vi "Making by Hot.vi"(0 "configuration file path":path caption="配置文件的路径", 1 "making by hot msic inf":T1) -> ()   [LabVIEW 2014]
uses:
  Ctl.xio/Making by Hot msic ctl.ctl
  SubVIS.xio/DataSocket/DataSocket_Tags.ctl
  Ctl.xio/part type.ctl
  <vilib>/Utility/file.llb/Read From Spreadsheet File (string).vi
panel:
  in  "SQL information":string
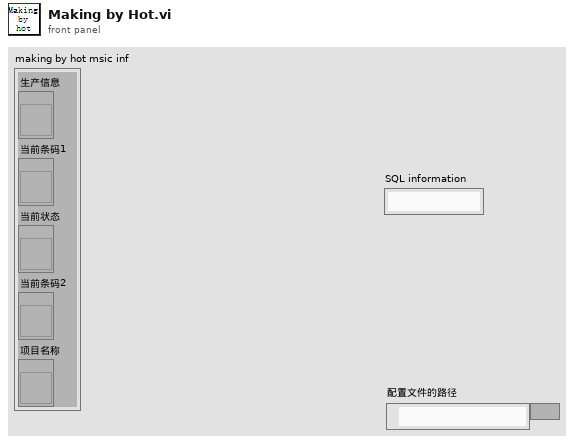
[diagram p1: front panel]
types:
  T1 = cluster{"生产信息":refnum<vi>, "当前条码1":refnum<vi>, "当前状态":refnum<vi>, "当前条码2":refnum<vi>, "项目名称":refnum<vi>}
  T2 = typedef "Making by Hot msic ctl.ctl" = cluster{"configuration file path":path, "DsOut":T3[], "BarCode1":string, "Hopper car information":cluster{"Hopper car code":string, "Hopper car No":string, "plate No":string}, "pallet.produced number":i32, "SQL information":string, "Database":string[], "Serial number":i32, "database path":path, "making by hot msic inf":cluster{"生产信息":refnum<vi>, "当前条码1":refnum<vi>, "当前状态":refnum<vi>, "当前条码2":refnum<vi>, "项目名称":refnum<vi>}, "scnner1 connect id":refnum<k5>, "scnner2 connect id":refnum<k5>, "scanner1 IP":string, "scanner2 IP":string, "BarCode2":string, "Heating process parameters":cluster{"heating start":string, "heating finish":string, "Heating time use":u32}, "part type":T4}
  T3 = typedef "DataSocket_Tags.ctl" = cluster{"Ds ID":refnum<k13>, "Tag":string}
  T4 = typedef "part type.ctl" = cluster{"项目号":string, "物料代码":string, "零件号":string, "供应商编码":string, "产线编码":string, "客户代码":string, "颜色代码":string, "托盘上限":i32, "加热温度":string, "加热时长":string, "EOL Stations":string}
  T5 = cluster{"Hopper car code":string, "Hopper car No":string, "plate No":string}
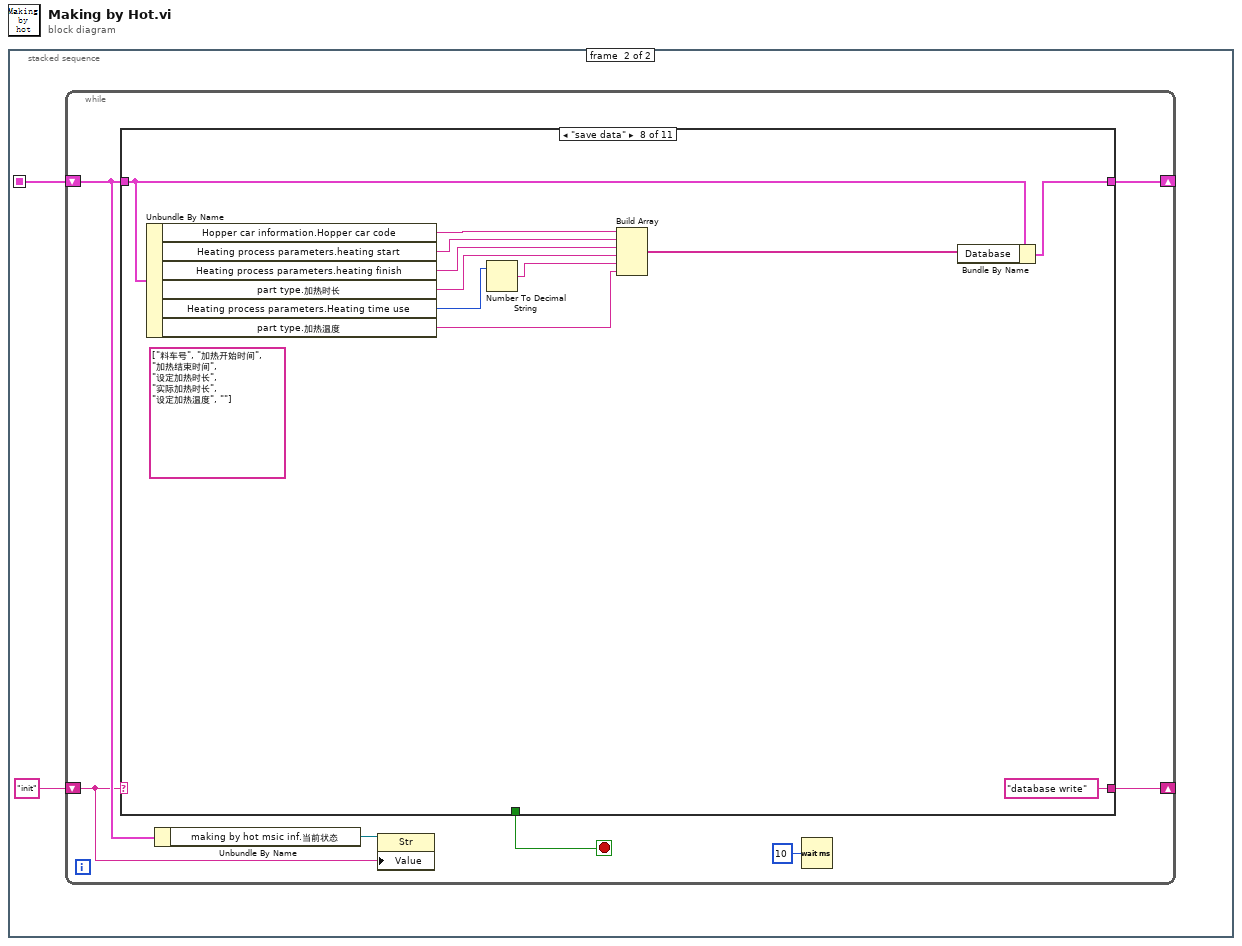
[diagram p0: block diagram]
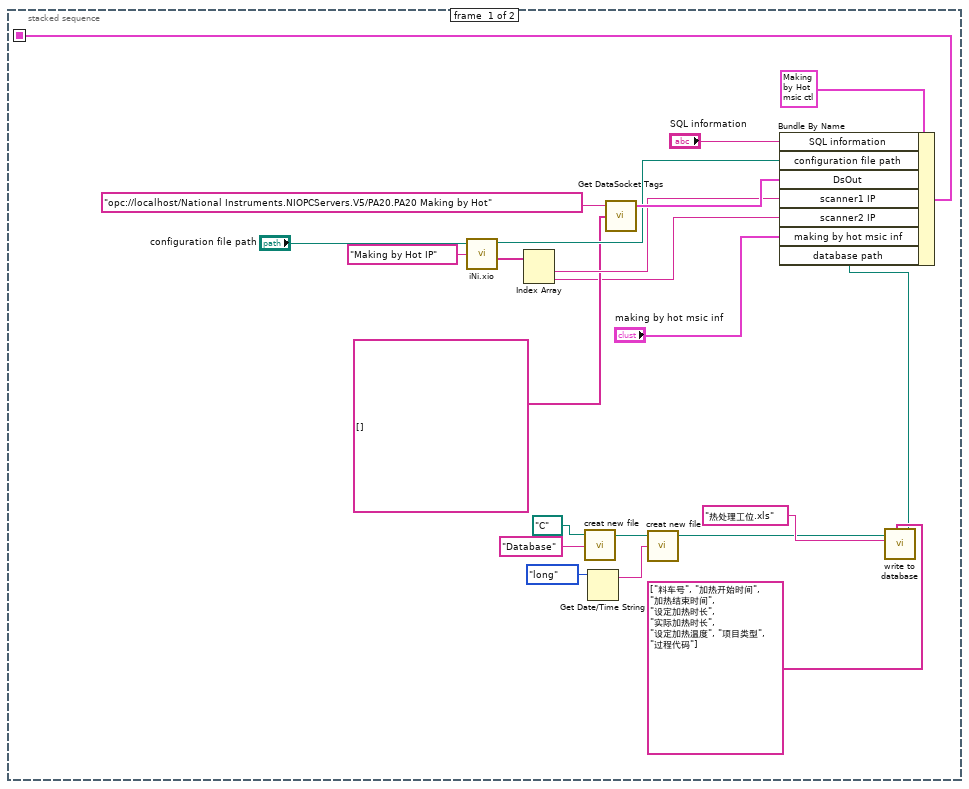
[diagram p2: hidden frame]
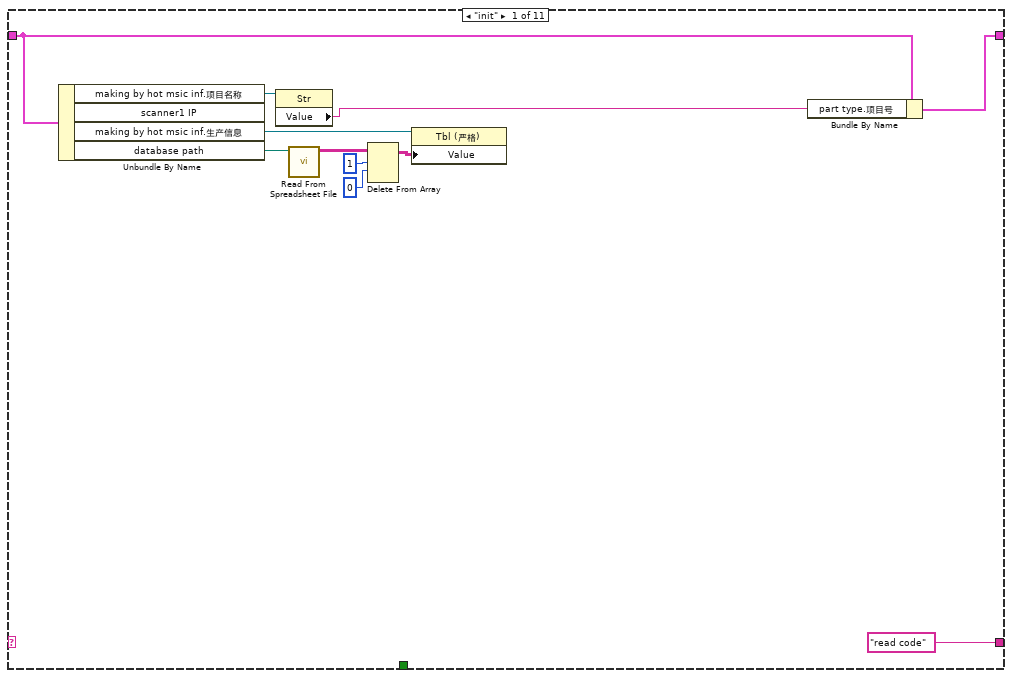
[diagram p3: hidden frame]
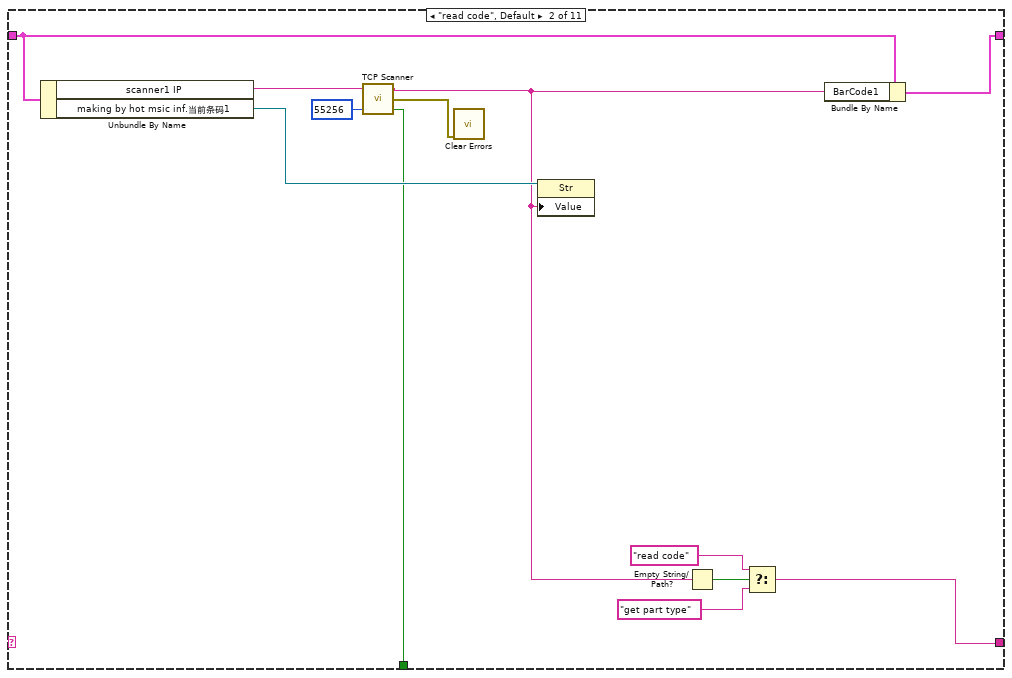
[diagram p4: hidden frame]
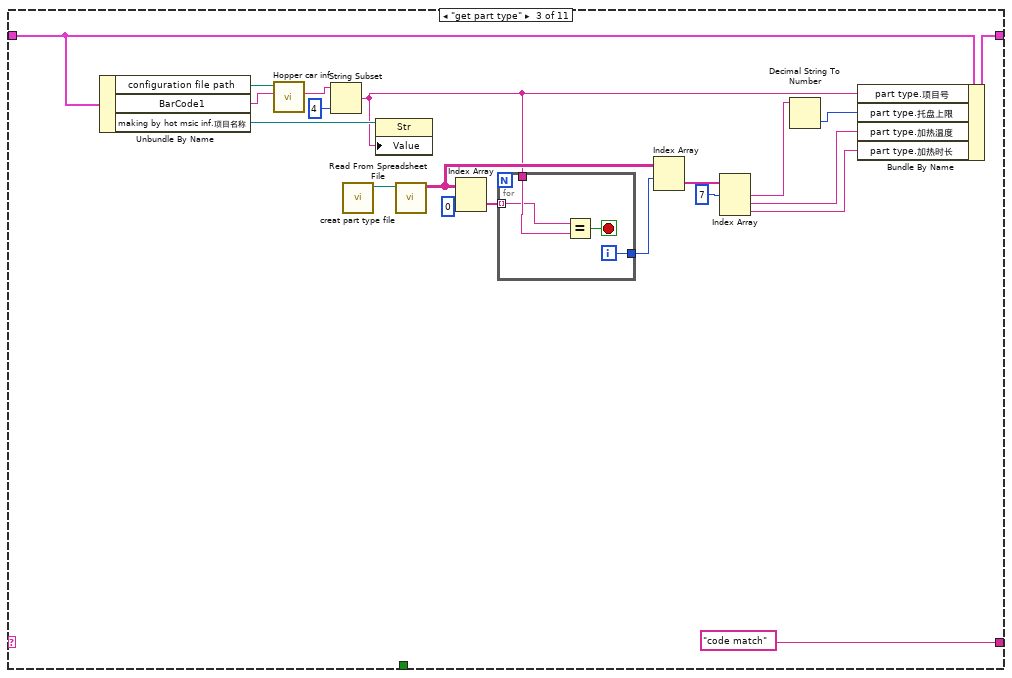
[diagram p5: hidden frame]
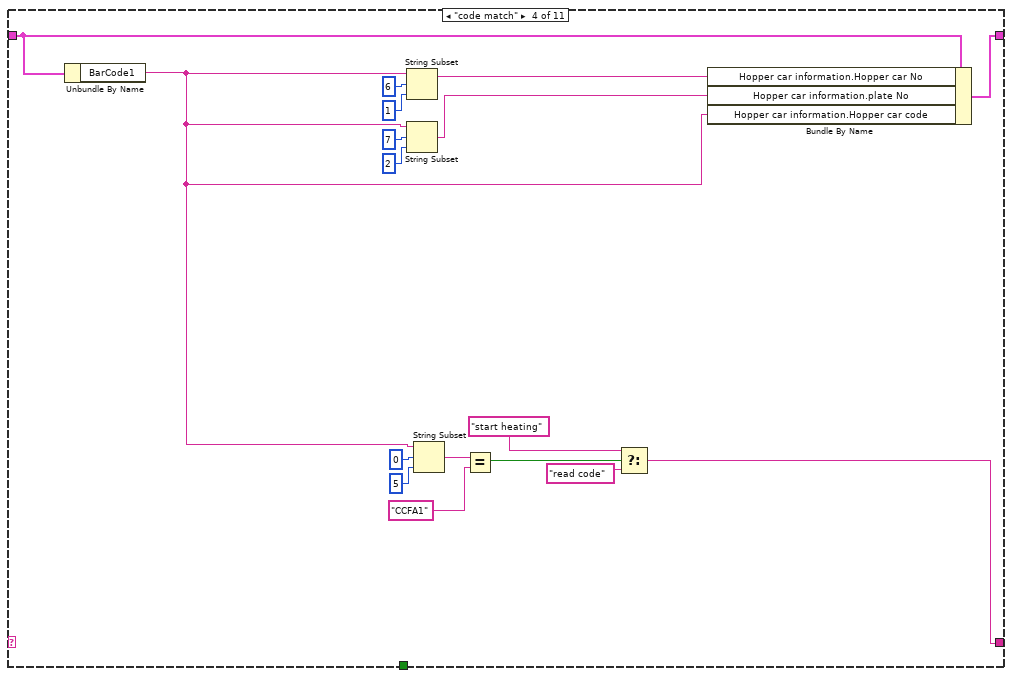
[diagram p6: hidden frame]
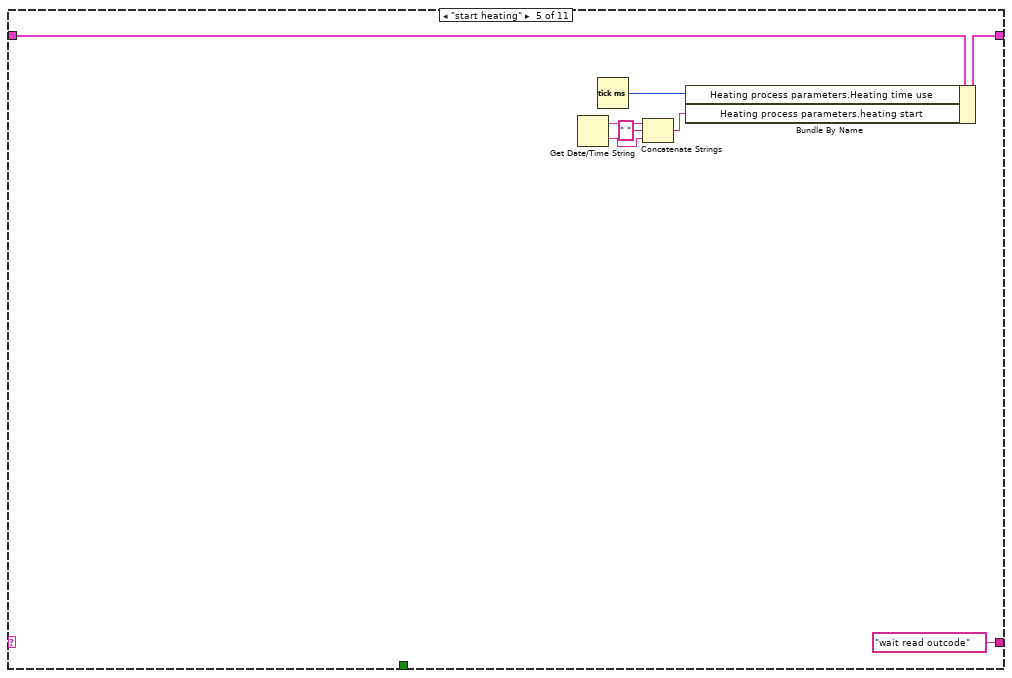
[diagram p7: hidden frame]
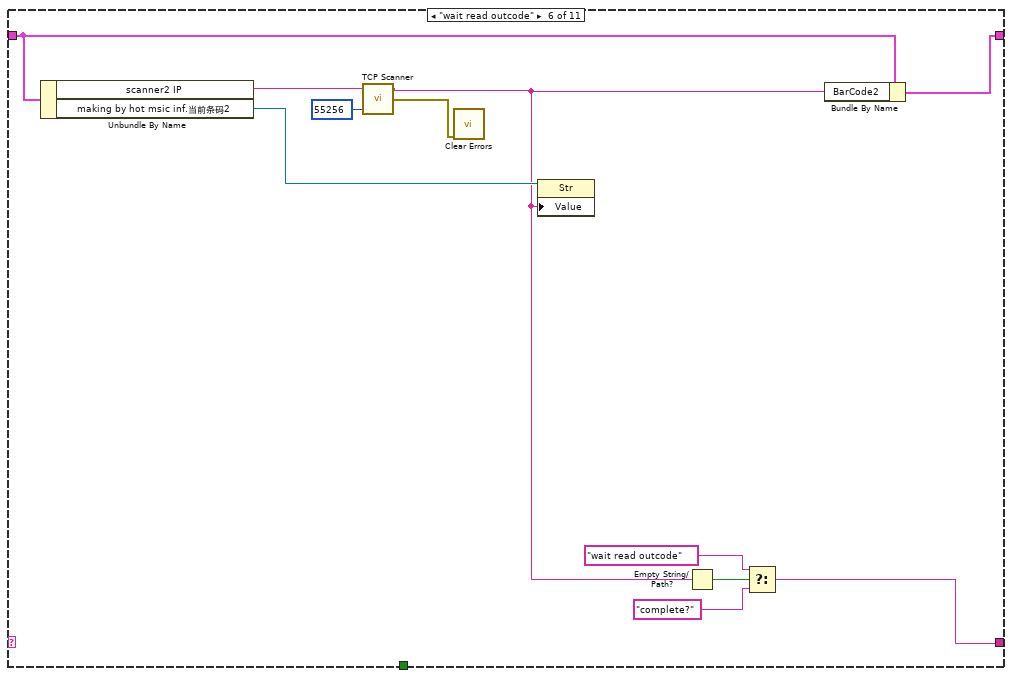
[diagram p8: hidden frame]
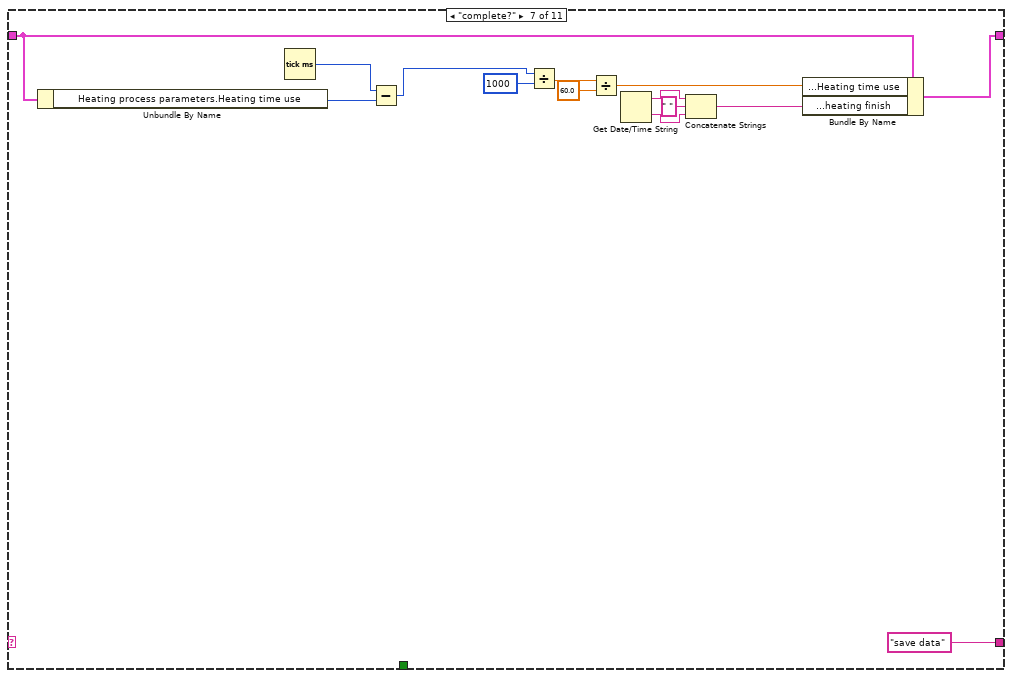
[diagram p9: hidden frame]
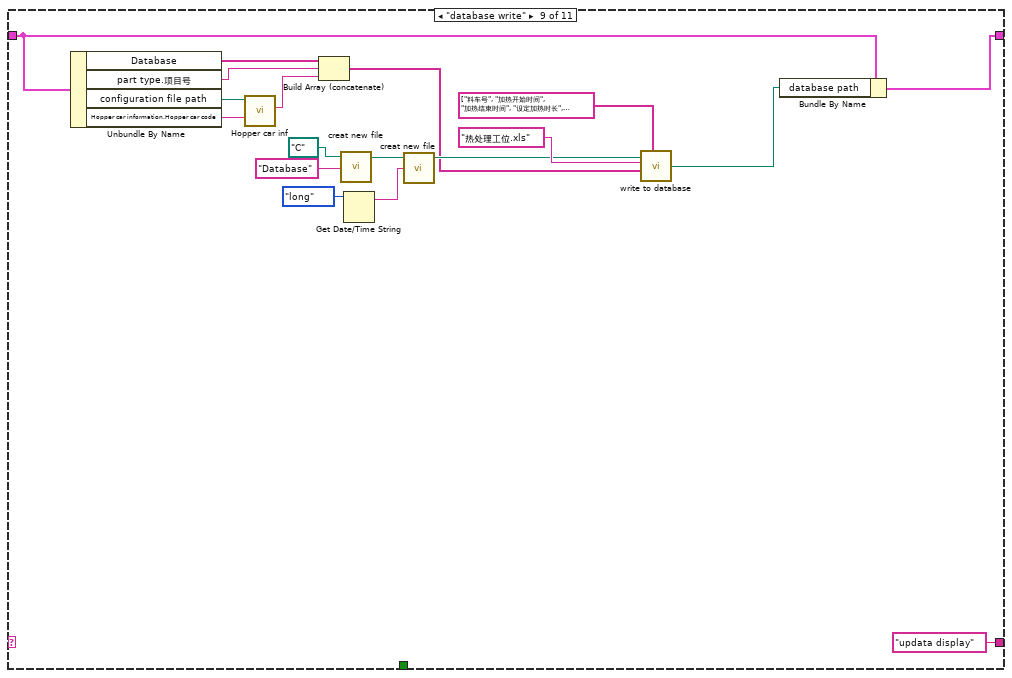
[diagram p10: hidden frame]
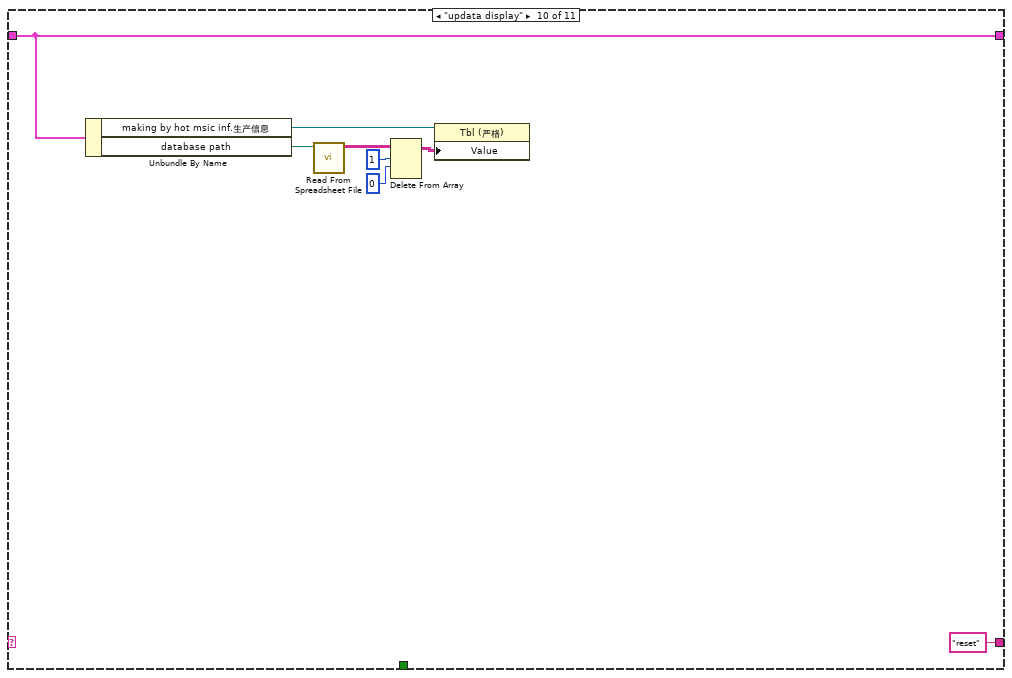
[diagram p11: hidden frame]
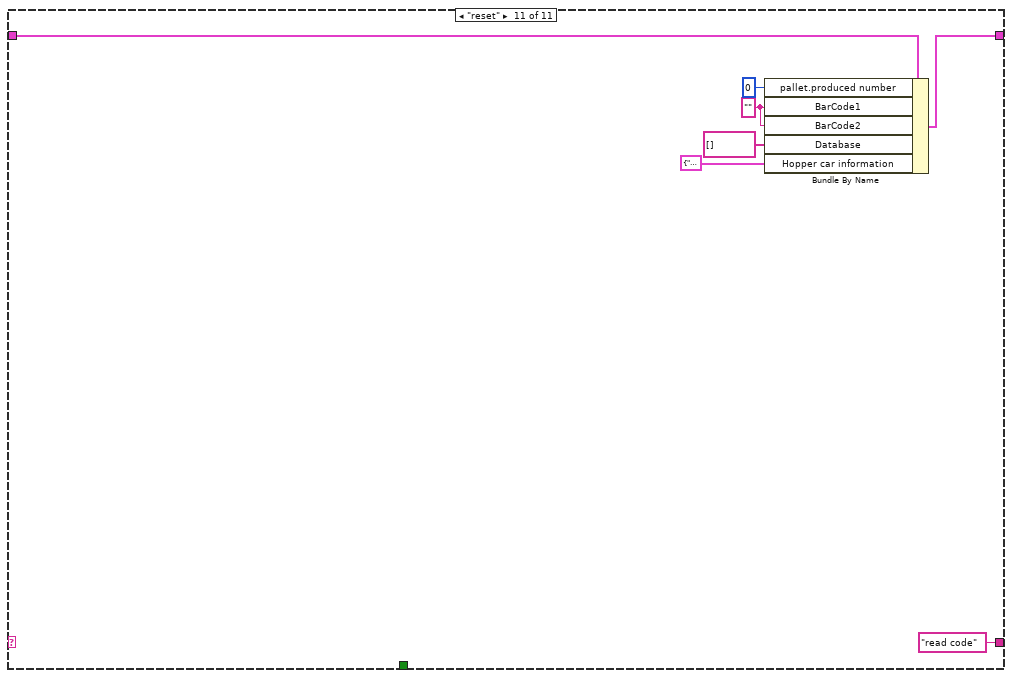
[diagram p12: hidden frame]
diagram:
  n1 = stacked-sequence {
    seq-local: [w10 _] -> [_ w23]
    frame #0 {
      n2 = call "iNi.xio.vi"("configuration file path"="configuration file path", "Sections"="Making by Hot IP") -> ("configuration file path"=w21:path, "Values"=w19:string[])  [unwired: 1 in, 3 out]
      n3 = Index Array(array=w19) -> (element #1=w18:string, element #2=w12:string)  [unwired: 2 in]
      n4 = call "creat new file.vi"("file name"="Database", "path"=path "C:/") -> ("created path"=w5:path)  [unwired: 1 in, 2 out]
      n5 = Get Date/Time String(date format (0)=enum16{"short", "long", "abbreviated"}."long" ("日期格式(0)")) -> (date string=w3:string)  [unwired: 2 in, 1 out]
      n6 = call "Get DataSocket Tags.vi"("All Tags"=string[] [], "URL"="opc://localhost/National Instruments.NIOPCServers.V5/PA20.PA20 Making by Hot") -> ("DsOut"=w22:T3[])  [unwired: 3 in]
      n7 = call "creat new file.vi"("file name"=w3, "path"=w5) -> ("created path"=w4:path)  [unwired: 1 in, 2 out]
      n8 = call "write to database.vi"("Header"=string[] ["料车号", "加热开始时间", "加热结束时间", "设定加热时长", "实际加热时长", "设定加热温度", "项目类型", "过程代码"], "file name"="热处理工位.xls", "path"=w4) -> ("new file path (Not A Path if cancelled)"=w2:path)  [unwired: 3 in]
      n9 = Bundle By Name(cluster=T2 {"configuration file path"=path "", "DsOut"=[], "BarCode1"="", "Hopper car information"={"Hopper car code"="", "Hopper car No"="", "plate No"=""}, "pallet.produced number"=0, "SQL information"="", "Database"=[], "Serial number"=0, "database path"=path "", "making by hot msic inf"={"生产信息"=refnum, "当前条码1"=refnum, "当前状态"=refnum, "当前条码2"=refnum, "项目名称"=refnum}, "scnner1 connect id"=refnum, "scnner2 connect id"=refnum, "scanner1 IP"="", "scanner2 IP"="", "BarCode2"="", "Heating process parameters"={"heating start"="", "heating finish"="", "Heating time use"=0}, "part type"={"项目号"="", "物料代码"="", "零件号"="", "供应商编码"="", "产线编码"="", "客户代码"="", "颜色代码"="", "托盘上限"=0, "加热温度"="", "加热时长"="", "EOL Stations"=""}} ("Making by Hot msic ctl"), "SQL information"="SQL information", "configuration file path"=w21, "DsOut"=w22, "scanner1 IP"=w18, "scanner2 IP"=w12, "making by hot msic inf"="making by hot msic inf", "database path"=w2) -> (w10:T2)
    }
    frame #1 {
      n10 = while {
        shift-right: [w31] -> _
        shift-left: w23 -> [w27]
        shift-right: [w30] -> _
        shift-left: "init" ("event") -> [w26]
        stop <- w25 stop-if-true
        n11 = case shown="\"save data\"" w26 {
          tunnel: w27 -> [w40 w52 w59 w80 w101 w112 w126 w138 w150 w162 w169]
          tunnel: [w42 w54 w74 w89 w103 w114 w121 w129 w151 w162 w171] -> w31
          tunnel: ["read code" w48 "code match" w87 "wait read outcode" ("event") w108 "save data" ("event") "database write" ("f") "updata display" ("f") "reset" ("f") "read code" ("f")] -> w30
          tunnel: [_ w43 _ _ _ _ _ _ _ _ _] -> w25
          frame "init" {
            n12 = Unbundle By Name(w40) -> ("making by hot msic inf.项目名称"=w39:refnum<vi>, "making by hot msic inf.生产信息"=w41:refnum<vi>, "database path"=w36:path)  [unwired: 1 out]
            n13 = property class="Str"(reference=w39) -> ("Value"=w38:string)  [unwired: 1 in, 2 out]
            n14 = call-poly <vilib>:"Read From Spreadsheet File.vi"("file path (dialog if empty)"=w36) -> ("all rows"=w33:string[][])  [unwired: 6 in, 4 out]
            n15 = Delete From Array(array=w33, length=1 ("长度"), index (row)=0 ("索引 (行)")) -> (array with subset deleted=w32:string[][])  [unwired: 1 in, 1 out]
            n16 = property class="Tbl (严格)"(reference=w41, "Value"=w32) -> ()  [unwired: 1 in, 2 out]
            n17 = Bundle By Name(cluster=w40, "part type.项目号"=w38) -> (w42:T2)
          }
          frame "read code", Default {
            n18 = Unbundle By Name(w52) -> ("scanner1 IP"=w46:string, "making by hot msic inf.当前条码1"=w53:refnum<vi>)
            n19 = call "TCP Scanner.vi"("Port（4001）"=u16 55256 ("远程端口或服务名称"), "ip"=w46) -> ("status"=w43:bool, "错误输出"=w44:errorcluster, "Barcode"=w45:string)  [unwired: 1 in]
            n20 = call <vilib>:"Clear Errors.vi"("error in (no error)"=w44) -> ()  [unwired: 5 in, 2 out]
            n21 = property class="Str"(reference=w53, "Value"=w45) -> ()  [unwired: 1 in, 2 out]
            n22 = Empty String/Path?(string/path=w45) -> (empty?=w51:bool)
            n23 = Select(t="read code" ("f"), s=w51, f="get part type") -> (s? t:f=w48:string)
            n24 = Bundle By Name(cluster=w52, "BarCode1"=w45) -> (w54:T2)
          }
          frame "get part type" {
            n25 = Unbundle By Name(w59) -> ("configuration file path"=w61:path, "BarCode1"=w60:string, "making by hot msic inf.项目名称"=w58:refnum<vi>)
            n26 = call "Hopper car inf.vi"("key"=w60, "path in"=w61) -> ("value out"=w57:string)  [unwired: 8 in, 1 out]
            n27 = String Subset(string=w57, length (rest)=4 ("长度（剩余）")) -> (substring=w55:string)  [unwired: 1 in]
            n28 = call "creat part type file.vi"() -> ("new file path (Not A Path if cancelled)"=w63:path)  [unwired: 11 in]
            n29 = property class="Str"(reference=w58, "Value"=w55) -> ()  [unwired: 1 in, 2 out]
            n30 = call-poly <vilib>:"Read From Spreadsheet File.vi"("file path (dialog if empty)"=w63) -> ("all rows"=w70:string[][])  [unwired: 6 in, 4 out]
            n31 = Index Array(array=w70, index (col)=0 ("禁用的索引 (列)")) -> (element=w72:string[])  [unwired: 1 in]
            n32 = for {
              tunnel: w72 -> [w75] mode=indexing
              tunnel: [w77] -> w69
              tunnel: w55 -> [w76]
              i -> [w77]
              stop <- w78 stop-if-true
              n33 = Equal?(x=w75, y=w76) -> (x = y?=w78:bool)
            }
            n34 = Index Array(array=w70, index (row)=w69) -> (element=w68:string[])  [unwired: 1 in]
            n35 = Index Array(array=w68, index #1=7 ("索引")) -> (element #1=w67:string, element #2=w65:string, element #3=w64:string)  [unwired: 2 in]
            n36 = Decimal String To Number(string=w67) -> (number=w66:i32)  [unwired: 2 in, 1 out]
            n37 = Bundle By Name(cluster=w59, "part type.项目号"=w55, "part type.托盘上限"=w66, "part type.加热温度"=w65, "part type.加热时长"=w64) -> (w74:T2)
          }
          frame "code match" {
            n38 = Unbundle By Name(w80) -> ("BarCode1"=w79:string)
            n39 = String Subset(string=w79, offset (0)=6 ("偏移量(0)"), length (rest)=1 ("长度（剩余）")) -> (substring=w82:string)
            n40 = String Subset(string=w79, offset (0)=7 ("偏移量(0)"), length (rest)=2 ("长度（剩余）")) -> (substring=w83:string)
            n41 = String Subset(string=w79, offset (0)=0 ("偏移量(0)"), length (rest)=5 ("长度（剩余）")) -> (substring=w84:string)
            n42 = Equal?(x=w84, y="CCFA1") -> (x = y?=w88:bool)
            n43 = Select(t="start heating" ("event"), s=w88, f="read code" ("event")) -> (s? t:f=w87:string)
            n44 = Bundle By Name(cluster=w80, "Hopper car information.Hopper car No"=w82, "Hopper car information.plate No"=w83, "Hopper car information.Hopper car code"=w79) -> (w89:T2)
          }
          frame "start heating" {
            n45 = Get Date/Time String() -> (date string=w99:string, time string=w97:string)  [unwired: 3 in]
            n46 = Tick Count (ms)() -> (millisecond timer value=w100:u32)
            n47 = Concatenate Strings(w99, " " ("字符串"), w97) -> (w96:string)
            n48 = Bundle By Name(cluster=w101, "Heating process parameters.Heating time use"=w100, "Heating process parameters.heating start"=w96) -> (w103:T2)
          }
          frame "wait read outcode" {
            n49 = Unbundle By Name(w112) -> ("scanner2 IP"=w106:string, "making by hot msic inf.当前条码2"=w113:refnum<vi>)
            n50 = call "TCP Scanner.vi"("Port（4001）"=u16 55256 ("远程端口或服务名称"), "ip"=w106) -> ("错误输出"=w104:errorcluster, "Barcode"=w105:string)  [unwired: 1 in, 1 out]
            n51 = call <vilib>:"Clear Errors.vi"("error in (no error)"=w104) -> ()  [unwired: 5 in, 2 out]
            n52 = property class="Str"(reference=w113, "Value"=w105) -> ()  [unwired: 1 in, 2 out]
            n53 = Empty String/Path?(string/path=w105) -> (empty?=w111:bool)
            n54 = Select(t="wait read outcode" ("f"), s=w111, f="complete?") -> (s? t:f=w108:string)
            n55 = Bundle By Name(cluster=w112, "BarCode2"=w105) -> (w114:T2)
          }
          frame "complete?" {
            n56 = Unbundle By Name(w126) -> ("Heating process parameters.Heating time use"=w127:u32)
            n57 = Tick Count (ms)() -> (millisecond timer value=w128:u32)
            n58 = Subtract(x=w128, y=w127) -> (x-y=w120:u32)
            n59 = Divide(x=w120, y=u32 1000) -> (x/y=w117:dbl)
            n60 = Divide(x=w117, y=60.0) -> (x/y=w115:dbl)
            n61 = Get Date/Time String() -> (date string=w122:string, time string=w124:string)  [unwired: 3 in]
            n62 = Concatenate Strings(w122, " " ("字符串"), w124) -> (w123:string)
            n63 = Bundle By Name(cluster=w126, "Heating process parameters.Heating time use"=w115, "Heating process parameters.heating finish"=w123) -> (w121:T2)
          }
          frame "save data" {
            (unwired) string[] ["料车号", "加热开始时间", "加热结束时间", "设定加热时长", "实际加热时长", "设定加热温度", ""] ("Header")
            n64 = Unbundle By Name(w138) -> ("Hopper car information.Hopper car code"=w137:string, "Heating process parameters.heating start"=w136:string, "Heating process parameters.heating finish"=w135:string, "part type.加热时长"=w134:string, "Heating process parameters.Heating time use"=w133:u32, "part type.加热温度"=w131:string)
            n65 = Number To Decimal String(number=w133) -> (decimal integer string=w132:string)  [unwired: 1 in]
            n66 = Build Array(w137, w136, w135, w134, w132, w131) -> (w130:string[])
            n67 = Bundle By Name(cluster=w138, "Database"=w130) -> (w129:T2)
          }
          frame "database write" {
            n68 = Unbundle By Name(w150) -> ("Database"=w146:string[], "part type.项目号"=w141:string, "configuration file path"=w144:path, "Hopper car information.Hopper car code"=w143:string)
            n69 = call "Hopper car inf.vi"("key"=w143, "path in"=w144) -> ("value out"=w142:string)  [unwired: 8 in, 1 out]
            n70 = Build Array (concatenate)(w146, w141, w142) -> (w145:string[])
            n71 = call "creat new file.vi"("file name"="Database", "path"=path "C:/") -> ("created path"=w149:path)  [unwired: 1 in, 2 out]
            n72 = Get Date/Time String(date format (0)=enum16{"short", "long", "abbreviated"}."long" ("日期格式(0)")) -> (date string=w147:string)  [unwired: 2 in, 1 out]
            n73 = call "creat new file.vi"("file name"=w147, "path"=w149) -> ("created path"=w148:path)  [unwired: 1 in, 2 out]
            n74 = call "write to database.vi"("Header"=string[] ["料车号", "加热开始时间", "加热结束时间", "设定加热时长", "实际加热时长", "设定加热温度", "项目类型", "过程代码"], "data in"=w145, "file name"="热处理工位.xls", "path"=w148) -> ("new file path (Not A Path if cancelled)"=w152:path)  [unwired: 2 in]
            n75 = Bundle By Name(cluster=w150, "database path"=w152) -> (w151:T2)
          }
          frame "updata display" {
            n76 = Unbundle By Name(w162) -> ("making by hot msic inf.生产信息"=w164:refnum<vi>, "database path"=w163:path)
            n77 = call-poly <vilib>:"Read From Spreadsheet File.vi"("file path (dialog if empty)"=w163) -> ("all rows"=w161:string[][])  [unwired: 6 in, 4 out]
            n78 = Delete From Array(array=w161, length=1 ("长度"), index (row)=0 ("索引 (行)")) -> (array with subset deleted=w158:string[][])  [unwired: 1 in, 1 out]
            n79 = property class="Tbl (严格)"(reference=w164, "Value"=w158) -> ()  [unwired: 1 in, 2 out]
          }
          frame "reset" {
            w168 = "" ("BarCode")
            n80 = Bundle By Name(cluster=w169, "pallet.produced number"=0, "BarCode1"=w168, "BarCode2"=w168, "Database"=string[] [], "Hopper car information"=T5 {"Hopper car code"="", "Hopper car No"="", "plate No"=""}) -> (w171:T2)
          }
        }
        n81 = Unbundle By Name(w27) -> ("making by hot msic inf.当前状态"=w28:refnum<vi>)
        n82 = property class="Str"(reference=w28, "Value"=w26) -> ()  [unwired: 1 in, 2 out]
        n83 = Wait (ms)(milliseconds to wait=u32 10 ("等待时间（毫秒）")) -> ()  [unwired: 1 out]
      }
    }
  }
